vi "CMD_MOVEREL.vi"(6 "Gantry in":refnum<class "Gantry.lvclass">, 8 "error in (no error)":errorcluster, 10 "Arguments":string[](array[string]), 11 "gScript Interpreter in":refnum<class "gScript Interpreter.lvclass">) -> (0 "error out":errorcluster, 3 "gScript Interpreter out":refnum<class "gScript Interpreter.lvclass">, 4 "Gantry out":refnum<class "Gantry.lvclass">)   [LabVIEW 2024, in "gScript Interpreter.lvclass"]
uses:
  gScript Interpreter.lvclass
  Shared Components/Gantry Class/Gantry.lvclass
  gScript Interpreter.lvclass/gScript Interpreter.ctl
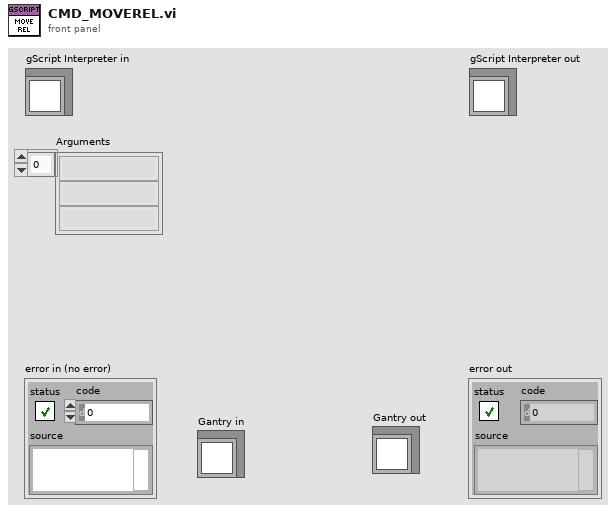
[diagram p1: front panel]
types:
  T1 = typedef "Memory Cell.ctl" = cluster{"type":T2, "x":dbl, "y":dbl, "z":dbl, "w":dbl}
  T2 = typedef "Memory Cell Type Enum.ctl" = enum16{"integer", "float", "vector", "rotation"}
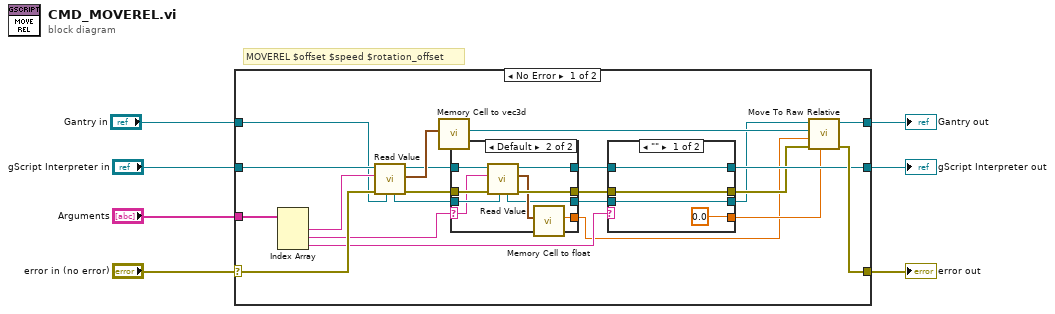
[diagram p0: block diagram]
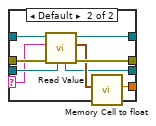
[diagram p2: hidden frame]
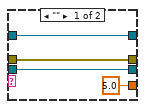
[diagram p3: hidden frame]
diagram:
  # "MOVEREL $offset $speed $rotation_offset"
  n1 = case shown="No Error" "error in (no error)" {
    selector: "error in (no error)" -> [w28 w58]
    tunnel: [w24 w58] -> w6
    tunnel: [w12 w57] -> w4
    tunnel: "gScript Interpreter in" -> [w29 w57]
    tunnel: "Arguments" -> [w27 _]
    tunnel: "Gantry in" -> [w19 w56]
    tunnel: [w23 w56] -> w1
    frame No Error {
      n2 = Index Array(array=w27) -> (element #1=w26:string, element #2=w17:string, element #3=w13:string)  [unwired: 3 in]
      n3 = call-dynamic "Read Value.vi"("Gantry in"=w19, "error in (no error)"=w28, "String in"=w26, "gScript Interpreter in"=w29) -> ("error out"=w25:errorcluster, "Memory Cell"=w22:T1, "gScript Interpreter out"=w20:refnum<class "gScript Interpreter.lvclass">, "Gantry out"=w18:refnum<class "Gantry.lvclass">)  [unwired: 4 in]
      n4 = call "Memory Cell to vec3d.vi"("Memory Cell"=w22) -> ("Vec3d out"=w21:refnum<class "Vec3d.lvclass">)  [unwired: 10 in]
      n5 = case shown="Default" w17 {
        selector: w17 -> [_ w47]
        tunnel: w25 -> [w45 w55]
        tunnel: w20 -> [w46 w54]
        tunnel: [w46 w53] -> w16
        tunnel: w18 -> [w44 w52]
        tunnel: [w45 w51] -> w15
        tunnel: [5.0 ("float out") w49] -> w9
        tunnel: [w44 w48] -> w14
        frame "" {
        }
        frame Default {
          n6 = call-dynamic "Read Value.vi"("Gantry in"=w52, "error in (no error)"=w55, "String in"=w47, "gScript Interpreter in"=w54) -> ("error out"=w51:errorcluster, "Memory Cell"=w50:T1, "gScript Interpreter out"=w53:refnum<class "gScript Interpreter.lvclass">, "Gantry out"=w48:refnum<class "Gantry.lvclass">)  [unwired: 4 in]
          n7 = call "Memory Cell to float.vi"("Memory Cell"=w50) -> ("float out"=w49:dbl)  [unwired: 10 in]
        }
      }
      n8 = case shown="\"\"" w13 {
        selector: w13 -> [_ w34]
        tunnel: w15 -> [w32 w42]
        tunnel: w16 -> [w33 w41]
        tunnel: [w33 w40] -> w12
        tunnel: w14 -> [w31 w39]
        tunnel: [w32 w38] -> w11
        tunnel: [0.0 w36] -> w10
        tunnel: [w31 w35] -> w8
        frame "" {
        }
        frame Default {
          n9 = call-dynamic "Read Value.vi"("Gantry in"=w39, "error in (no error)"=w42, "String in"=w34, "gScript Interpreter in"=w41) -> ("error out"=w38:errorcluster, "Memory Cell"=w37:T1, "gScript Interpreter out"=w40:refnum<class "gScript Interpreter.lvclass">, "Gantry out"=w35:refnum<class "Gantry.lvclass">)  [unwired: 4 in]
          n10 = call "Memory Cell to float.vi"("Memory Cell"=w37) -> ("float out"=w36:dbl)  [unwired: 10 in]
        }
      }
      n11 = call-dynamic "Move To Raw Relative.vi"("Rotation Angle"=w10, "error in"=w11, "Speed(mm/s)"=w9, "Delta"=w21, "Gantry in"=w8) -> ("error out"=w24:errorcluster, "Gantry out"=w23:refnum<class "Gantry.lvclass">)  [unwired: 5 in]
    }
    frame Error {
    }
  }
  "error out" <- w6
  "gScript Interpreter out" <- w4
  "Gantry out" <- w1
